vi "Open Motors V.3.0.vi"   [LabVIEW 2017]
uses:
  <vilib>/Rock Robotics/WPI/RobotDrive/WPI_RobotDriveOpen4MotorWithExistingMotors.vi
types:
  T1 = typedef "WPI_MotorControlDeviceRef.ctl" = cluster{"DeviceStatus":errorcluster, "Type":T2, "PWM":cluster{"PWM Channel":T3, "DeadBand":T4}, "CAN":cluster{"Device Number":u8, "SetOutput VI Ref":variant, "GetOutput VI Ref":variant, "Enable VI Ref":variant, "Disable VI Ref":variant, "Data":variant}, "Invert":bool, "DIO PWM":cluster{"PWM \"Enable\" Channel":T3, "DIOChannel":T5, "PWM Rate":dbl}}
  T2 = typedef "WPI_MotorControlType.ctl" = enum16{"PWM", "CAN", "DIO PWM"}
  T3 = typedef "FPGA_DIOPWMChannel.ctl" = enum8{"PWM 0", "PWM 1", "PWM 2", "PWM 3", "PWM 4", "PWM 5", "PWM 6", "PWM 7", "PWM 8", "PWM 9", "PWM MXP 0", "PWM MXP 1", "PWM MXP 2", "PWM MXP 3", "PWM MXP 4", "PWM MXP 5", "PWM MXP 6", "PWM MXP 7", "PWM MXP 8", "PWM MXP 9", "Invalid"}
  T4 = typedef "WPI_PWMDeadband.ctl" = cluster{"Name":string, "maxPositivePwm":i32, "minPositivePwm":i32, "centerPwm":i32, "maxNegativePwm":i32, "minNegativePwm":i32, "angularRange":u16}
  T5 = typedef "FPGA_DIOChannel.ctl" = enum8{"DIO 0", "DIO 1", "DIO 2", "DIO 3", "DIO 4", "DIO 5", "DIO 6", "DIO 7", "DIO 8", "DIO 9", "DIO MXP 0", "DIO MXP 1", "DIO MXP 2", "DIO MXP 3", "DIO MXP 4", "DIO MXP 5", "DIO MXP 6", "DIO MXP 7", "DIO MXP 8", "DIO MXP 9", "DIO MXP 10", "DIO MXP 11", "DIO MXP 12", "DIO MXP 13", "DIO MXP 14", "DIO MXP 15", "SPI Port CS1", "SPI Port CS2", "SPI Port CS3", "SPI Port MISO", "SPI Port MOSI", "Invalid"}
  T6 = typedef "WPI_RobotDriveDevRef.ctl" = cluster{"DevStatus":errorcluster, "Motors[]":T1[], "Square Inputs":bool, "Max Output":dbl}
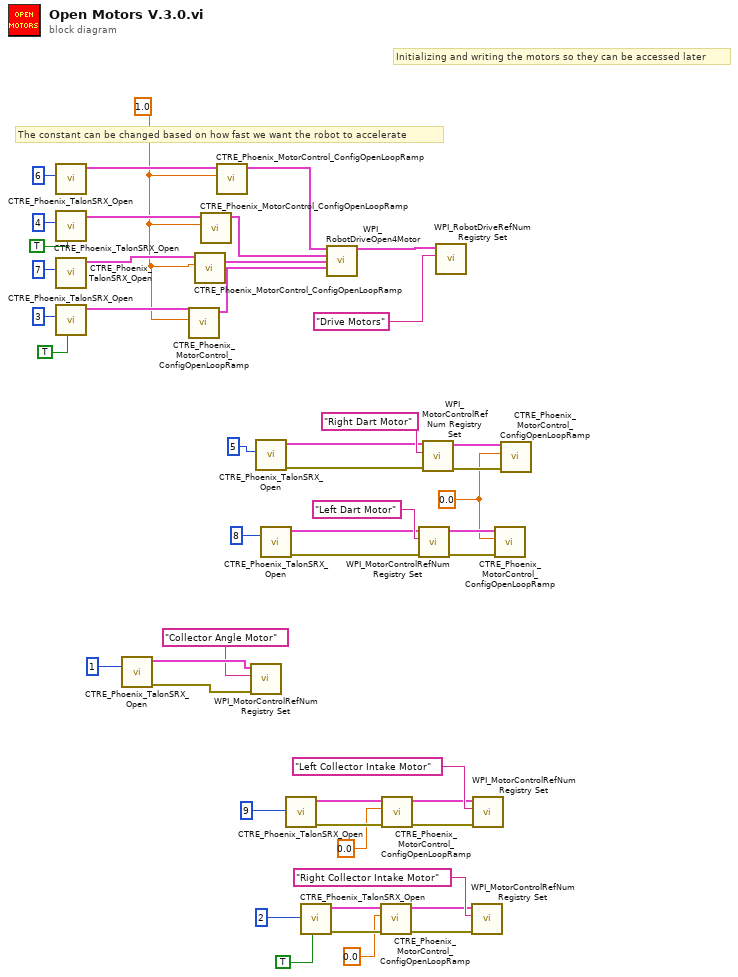
[diagram p0: block diagram]
diagram:
  w12 = 1.0
  w28 = 0.0
  # "The constant can be changed based on how fast we want the robot to accelerate"
  # "Initializing and writing the motors so they can be accessed later"
  n1 = call "CTRE_Phoenix_TalonSRX_Open.vi"("Device Number"=u8 6) -> ("CAN Talon SRX Ref"=w24:T1)  [unwired: 9 in, 1 out]
  n2 = call "CTRE_Phoenix_TalonSRX_Open.vi"("Invert"=TRUE, "Device Number"=u8 4) -> ("CAN Talon SRX Ref"=w21:T1)  [unwired: 8 in, 1 out]
  n3 = call "CTRE_Phoenix_TalonSRX_Open.vi"("Device Number"=u8 7) -> ("CAN Talon SRX Ref"=w18:T1)  [unwired: 9 in, 1 out]
  n4 = call "CTRE_Phoenix_TalonSRX_Open.vi"("Invert"=TRUE, "Device Number"=u8 3) -> ("CAN Talon SRX Ref"=w22:T1)  [unwired: 8 in, 1 out]
  n5 = call "CTRE_Phoenix_TalonSRX_Open.vi"("Device Number"=1) -> ("error out"=w27:errorcluster, "CAN Talon SRX Ref"=w26:T1)  [unwired: 9 in]
  n6 = call "CTRE_Phoenix_MotorControl_ConfigOpenLoopRamp.vi"("secondsFromNeutralToFull"=w12, "PhoenixMotorControlDevRef"=w22) -> ("PhoenixMotorControlDevRef"=w19:T1)  [unwired: 8 in, 1 out]
  n7 = call "CTRE_Phoenix_MotorControl_ConfigOpenLoopRamp.vi"("secondsFromNeutralToFull"=w12, "PhoenixMotorControlDevRef"=w18) -> ("PhoenixMotorControlDevRef"=w17:T1)  [unwired: 8 in, 1 out]
  n8 = call "CTRE_Phoenix_MotorControl_ConfigOpenLoopRamp.vi"("secondsFromNeutralToFull"=w12, "PhoenixMotorControlDevRef"=w21) -> ("PhoenixMotorControlDevRef"=w20:T1)  [unwired: 8 in, 1 out]
  n9 = call "CTRE_Phoenix_MotorControl_ConfigOpenLoopRamp.vi"("secondsFromNeutralToFull"=w12, "PhoenixMotorControlDevRef"=w24) -> ("PhoenixMotorControlDevRef"=w23:T1)  [unwired: 8 in, 1 out]
  n10 = call <vilib>:"WPI_MotorControlRefNum Registry Set.vi"("error in (no error)"=w27, "refnum name"="Collector Angle Motor", "MotorControlDevRef"=w26) -> ()  [unwired: 7 in, 2 out]
  n11 = call "CTRE_Phoenix_TalonSRX_Open.vi"("Device Number"=u8 5) -> ("error out"=w35:errorcluster, "CAN Talon SRX Ref"=w36:T1)  [unwired: 9 in]
  n12 = call "CTRE_Phoenix_TalonSRX_Open.vi"("Device Number"=u8 8) -> ("error out"=w33:errorcluster, "CAN Talon SRX Ref"=w34:T1)  [unwired: 9 in]
  n13 = call "CTRE_Phoenix_TalonSRX_Open.vi"("Device Number"=9) -> ("error out"=w7:errorcluster, "CAN Talon SRX Ref"=w10:T1)  [unwired: 9 in]
  n14 = call "CTRE_Phoenix_TalonSRX_Open.vi"("Invert"=TRUE, "Device Number"=2) -> ("error out"=w3:errorcluster, "CAN Talon SRX Ref"=w6:T1)  [unwired: 8 in]
  n15 = call-poly <vilib>:"WPI_RobotDriveOpen4Motor.vi"("Rear Left Motor Dev Ref"=w23, "Rear Right Motor Dev Ref"=w20, "Front Left Motor Dev Ref"=w17, "Front Right Motor Dev Ref"=w19) -> ("RobotDriveDevRef"=w11:T6)  [unwired: 10 in, 1 out]
  n16 = call "CTRE_Phoenix_MotorControl_ConfigOpenLoopRamp.vi"("error in (no error)"=w3, "secondsFromNeutralToFull"=0.0, "PhoenixMotorControlDevRef"=w6) -> ("error out"=w4:errorcluster, "PhoenixMotorControlDevRef"=w5:T1)  [unwired: 7 in]
  n17 = call "CTRE_Phoenix_MotorControl_ConfigOpenLoopRamp.vi"("error in (no error)"=w7, "secondsFromNeutralToFull"=0.0, "PhoenixMotorControlDevRef"=w10) -> ("error out"=w8:errorcluster, "PhoenixMotorControlDevRef"=w9:T1)  [unwired: 7 in]
  n18 = call <vilib>:"WPI_MotorControlRefNum Registry Set.vi"("error in (no error)"=w33, "refnum name"="Left Dart Motor", "MotorControlDevRef"=w34) -> ("error out"=w29:errorcluster, "MotorControlDevRef"=w30:T1)  [unwired: 7 in]
  n19 = call <vilib>:"WPI_MotorControlRefNum Registry Set.vi"("error in (no error)"=w35, "refnum name"="Right Dart Motor", "MotorControlDevRef"=w36) -> ("error out"=w31:errorcluster, "MotorControlDevRef"=w32:T1)  [unwired: 7 in]
  n20 = call <vilib>:"WPI_RobotDriveRefNum Registry Set.vi"("refnum name"="Drive Motors", "RobotDriveDevRef"=w11) -> ()  [unwired: 8 in, 2 out]
  n21 = call <vilib>:"WPI_MotorControlRefNum Registry Set.vi"("error in (no error)"=w4, "refnum name"="Right Collector Intake Motor", "MotorControlDevRef"=w5) -> ()  [unwired: 7 in, 2 out]
  n22 = call <vilib>:"WPI_MotorControlRefNum Registry Set.vi"("error in (no error)"=w8, "refnum name"="Left Collector Intake Motor", "MotorControlDevRef"=w9) -> ()  [unwired: 7 in, 2 out]
  n23 = call "CTRE_Phoenix_MotorControl_ConfigOpenLoopRamp.vi"("error in (no error)"=w29, "secondsFromNeutralToFull"=w28, "PhoenixMotorControlDevRef"=w30) -> ()  [unwired: 7 in, 2 out]
  n24 = call "CTRE_Phoenix_MotorControl_ConfigOpenLoopRamp.vi"("error in (no error)"=w31, "secondsFromNeutralToFull"=w28, "PhoenixMotorControlDevRef"=w32) -> ()  [unwired: 7 in, 2 out]
